vi "FormatAssignment.vi"(1 "value":string, 2 "name":string) -> (0 "python assignment":string)   [LabVIEW 2014, in "Python Functions.lvlib"]
uses:
  Python Functions.lvlib
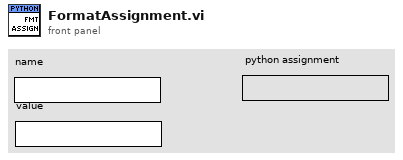
[diagram p1: front panel]
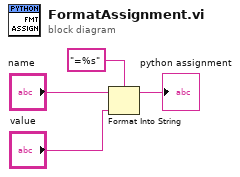
[diagram p0: block diagram]
diagram:
  n1 = Format Into String(format string="=%s", initial string="name", "value") -> (resulting string=→"python assignment":string)  [unwired: 1 in, 1 out]
